vi "comms_Serial_Open_nocommand.vi"(8 "error in (no error)":errorcluster, 9 "Serial Settings in":T1, 11 "VISA Refnum in":refnum<visa-resource-name>) -> (0 "error out":errorcluster, 2 "Data Out":string, 3 "VISA Refnum out":refnum<visa-resource-name>)   [LabVIEW 2018]
uses:
  <vilib>/Instr/_visa.llb/VISA Configure Serial Port (Instr).vi
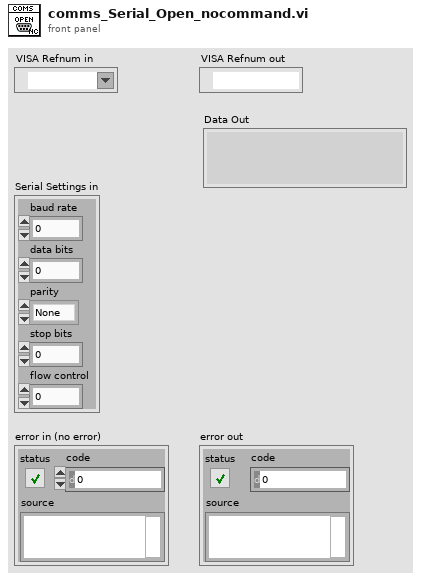
[diagram p1: front panel]
types:
  T1 = cluster{"baud rate":u32, "data bits":u16, "parity":enum16{"None", "Odd", "Even", "Mark", "Space"}, "stop bits":u16, "flow control":u16}
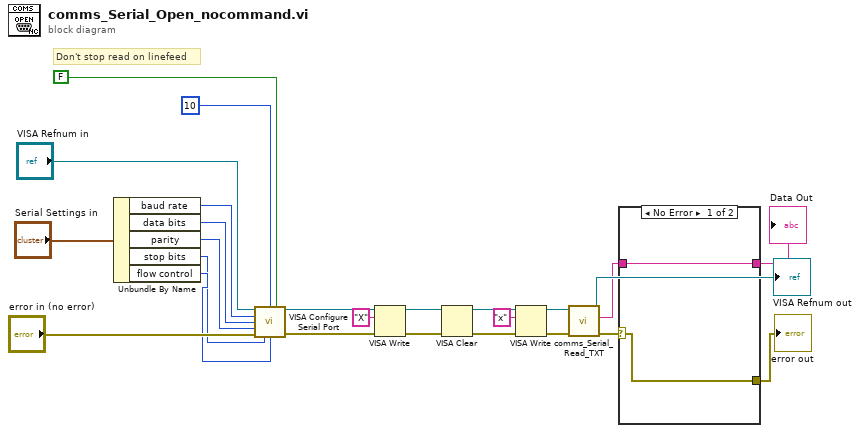
[diagram p0: block diagram]
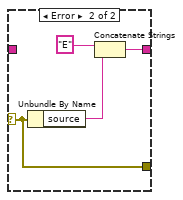
[diagram p2: hidden frame]
diagram:
  # "Don't stop read on linefeed"
  n1 = Unbundle By Name("Serial Settings in") -> ("baud rate"=w20:u32, "data bits"=w19:u16, "parity"=w18:enum16{"None", "Odd", "Even", "Mark", "Space"}, "stop bits"=w17:u16, "flow control"=w23:u16)
  n2 = call-poly "VISA Configure Serial Port"("VISA resource name"="VISA Refnum in", "termination char\n(0xA = '\\n' = LF)"=u8 10 ("Termination Character"), "Enable Termination\nChar (T)"=FALSE ("End Read on Termination Character?"), "baud rate (9600)"=w20, "data bits (8)"=w19, "parity (0:none)"=w18, "error in (no error)"="error in (no error)", "stop bits (10: 1 bit)"=w17, "flow control (0:none)"=w23) -> ("VISA resource name out"=w10:refnum<visa-resource-name>, "error out"=w9:errorcluster)  [unwired: 1 in, 4 out]
  n3 = VISA Write(VISA resource name=w10, write buffer="X", error in (no error)=w9) -> (VISA resource name out=w6:refnum<visa-resource-name>, error out=w7:errorcluster)  [unwired: 1 out]
  n4 = VISA Clear(VISA resource name=w6, error in (no error)=w7) -> (VISA resource name out=w3:refnum<visa-resource-name>, error out=w5:errorcluster)
  n5 = VISA Write(VISA resource name=w3, write buffer="x", error in (no error)=w5) -> (VISA resource name out=w2:refnum<visa-resource-name>, error out=w4:errorcluster)  [unwired: 1 out]
  n6 = call "comms_Serial_Read_TXT.vi"("error in"=w4, "VISA resource in"=w2) -> ("error out"=w14:errorcluster, "Data Out"=w12:string, "VISA resource Out"=→"VISA Refnum out":refnum<visa-resource-name>)  [unwired: 6 in, 1 out]
  n7 = case shown="No Error" w14 {
    selector: w14 -> [w27 w31]
    tunnel: [w27 w31] -> w13
    tunnel: w12 -> [w26 _]
    tunnel: [w26 w30] -> w11
    frame No Error {
    }
    frame Error {
      n8 = Unbundle By Name(w31) -> ("source"=w29:string)
      n9 = Concatenate Strings("E", w29) -> (w30:string)
    }
  }
  "error out" <- w13
  "Data Out" <- w11
